vi "Locating Sensor.vi"() -> ()   [LabVIEW 2016]
uses:
  Classes/Workspace/Workspace.ctl
  Classes/Workspace/Component/Component Tray.lvclass
  Classes/Controller/Controller.lvclass
  Classes/Workspace/Fixture.lvclass
panel:
  out "Workspace":T1
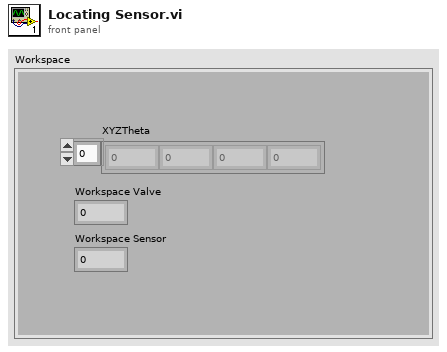
[diagram p1: front panel]
types:
  T1 = typedef "Fixture.lvclass/Workspace.ctl" = cluster{"XYZTheta":dbl[], "Workspace Valve":i32, "Workspace Sensor":i32}
  T2 = typedef "Controller.lvclass/Controllers.ctl" = cluster{"I-O.lvclass":refnum<class "I-O.lvclass">, "Motion.lvclass":refnum<class "Motion.lvclass">, "Dispenser.lvclass":refnum<class "Dispenser.lvclass">}
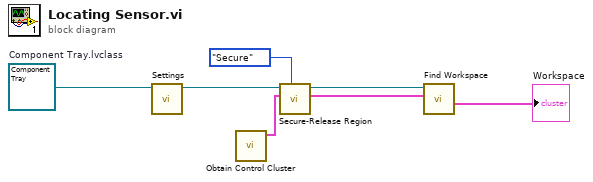
[diagram p0: block diagram]
diagram:
  w2 = refnum<class "Component Tray.lvclass"> refnum  # Component Tray.lvclass
  n1 = call-dynamic "Settings.vi"("Component in"=w2) -> ("Component out"=w7:refnum<class "Component Tray.lvclass">)  [unwired: 9 in, 1 out]
  n2 = call "Obtain Control Cluster.vi"() -> ("Control Out"=w6:T2)  [unwired: 11 in]
  n3 = call-dynamic "Secure-Release Region.vi"("Action"=enum16{"Secure", "Release"}."Secure", "Control In"=w6, "Component in"=w7) -> ("Control Out"=w4:T2, "Component out"=w5:refnum<class "Component Tray.lvclass">)  [unwired: 6 in, 1 out]
  n4 = call-dynamic "Find Workspace.vi"("Control In"=w4, "Component.lvclass"=w5) -> ("Workspace"=→"Workspace":T1)  [unwired: 6 in, 3 out]
